vi "Test PC Sensor.vi"() -> ()   [LabVIEW 2019, in "Temperhum.PCSensor.lvclass"]
uses:
  Temperhum.PCSensor.lvclass
panel:
  in  "stop":bool
  out "Temp Chart":dbl(graph)
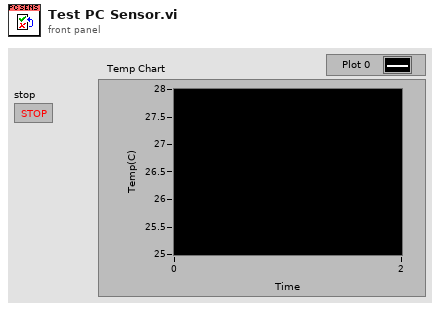
[diagram p1: front panel]
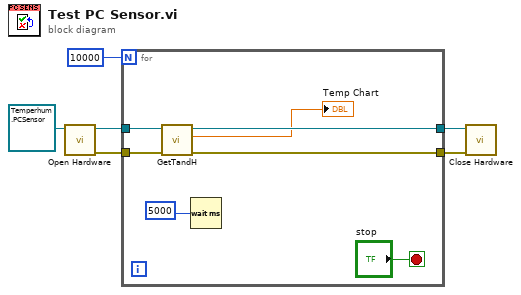
[diagram p0: block diagram]
diagram:
  n1 = call-dynamic "Open Hardware.vi"("Instrument.FrameworkTemplate"=refnum<class "Temperhum.PCSensor.lvclass"> refnum) -> ("error out"=w4:errorcluster, "Instrument.FrameworkTemplate out"=w5:refnum<class "Temperhum.PCSensor.lvclass">)  [unwired: 9 in]
  n2 = for {
    N: 10000 -> [_]
    tunnel: w5 -> [w12]
    tunnel: w4 -> [w11]
    tunnel: [w10] -> w3
    tunnel: [w9] -> w2
    stop <- "stop" stop-if-true
    n3 = call-dynamic "GetTandH.vi"("error in (no error)"=w11, "Temperhum.PCSensor in"=w12) -> ("error out"=w9:errorcluster, "Temperature (K)"=→"Temp Chart":dbl, "Temperhum.PCSensor out"=w10:refnum<class "Temperhum.PCSensor.lvclass">)  [unwired: 6 in, 1 out]
    n4 = Wait (ms)(milliseconds to wait=u32 5000 ("millisecond timer value")) -> ()  [unwired: 1 out]
  }
  n5 = call-dynamic "Close Hardware.vi"("error in (no error)"=w2, "Instrument.FrameworkTemplate"=w3) -> ()  [unwired: 8 in, 2 out]
